vi "Check for Fresh Message.vi"(8 "error in":errorcluster, 11 "Handle Stop Message in":refnum<class "Handle Stop Message.lvclass">) -> (0 "error out":errorcluster, 1 "Enqueuer":refnum<class "Message Enqueuer.lvclass">, 2 "Enqueuer not Valid":bool, 3 "Handle Stop Message out":refnum<class "Handle Stop Message.lvclass">)   [LabVIEW 2014, in "Handle Stop Message.lvclass"]
doc: "This method is a dynamic method that \n1) checks for a good connection to the shared variable. If it is not present, then it attempts to connect If a connection is not available, then this VI will do nothing.\n2) Check the state of the enqueuer. If the state is no good, return with this indication and do nothing.\n2) If the connection is good, check to see if the current shared variable state has changed.\n3) If the state has changed, pump the message into the appropriate enqueuer."
uses:
  Handle Stop Message.lvclass
  <vilib>/ActorFramework/Message Enqueuer/Message Enqueuer.lvclass
  <vilib>/ActorFramework/Message Enqueuer/Message Enqueuer.lvclass/Message Enqueuer.ctl
  <vilib>/ActorFramework/Message Enqueuer/Enqueue.vi
  <vilib>/ActorFramework/Message Priority Queue/Priority Enqueue.vi
  Network Command Processor.lvclass
  <vilib>/ActorFramework/Stop Msg/Stop Msg.lvclass
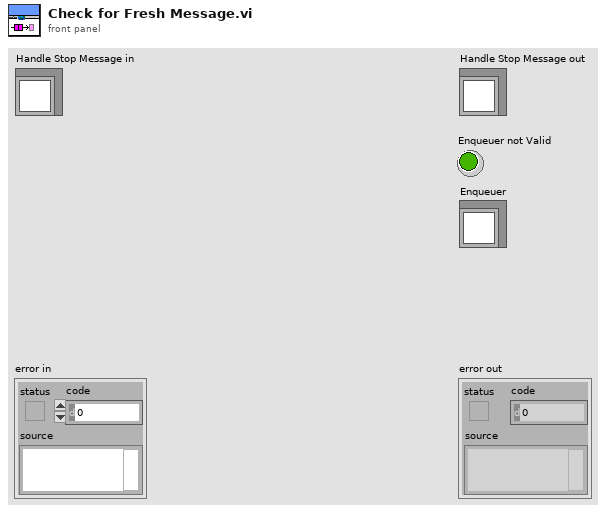
[diagram p1: front panel]
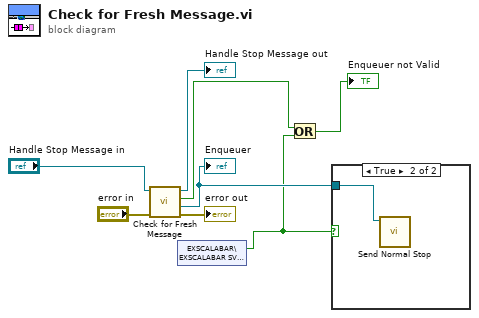
[diagram p0: block diagram]
diagram:
  n1 = call-parent "Check for Fresh Message.vi"("error in"="error in", "Network Command Processor in"="Handle Stop Message in") -> ("error out"=→"error out":errorcluster, "Enqueuer"=w4:refnum<class "Message Enqueuer.lvclass">, "Enqueuer not Valid"=w3:bool, "Network Command Processor out"=→"Handle Stop Message out":refnum<class "Handle Stop Message.lvclass">)  [unwired: 6 in]
  "Enqueuer" <- w4
  n2 = shared-variable "EXSCALABAR\\EXSCALABAR SV.lvlib\\Stop"() -> (w2:bool)  [unwired: 1 in, 1 out]
  n3 = Or(x=w3, y=w2) -> (x .or. y?=→"Enqueuer not Valid":bool)
  n4 = case shown="True" w2 {
    tunnel: w4 -> [_ w9]
    frame False {
    }
    frame True {
      n5 = call <vilib>:"Send Normal Stop.vi"("Message Enqueuer"=w9) -> ()  [unwired: 10 in, 1 out]
    }
  }
